vi "DownloadFile.vi"(8 "error in":errorcluster, 11 "Downloader in":refnum<class "Downloader.lvclass">) -> (0 "error out":errorcluster, 3 "Downloader out":refnum<class "Downloader.lvclass">)   [LabVIEW 2014, in "Downloader.lvclass"]
uses:
  Downloader.lvclass
  Downloader.lvclass/Downloader.ctl
  MessageBox/MessageBox.lvclass
  Websocket/Websocket.lvlib
  Download/RasPiDownloader.lvlib
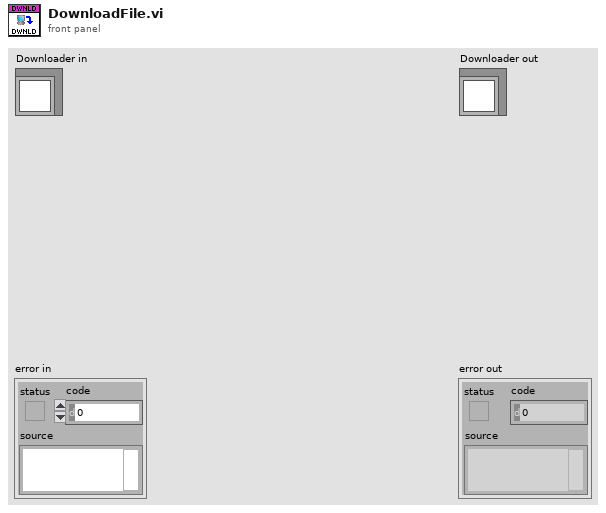
[diagram p1: front panel]
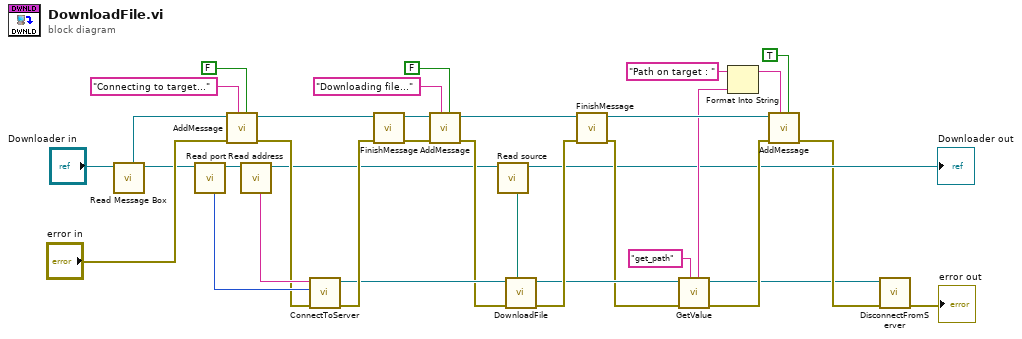
[diagram p0: block diagram]
diagram:
  n1 = call "Read Message Box.vi"("Downloader in"="Downloader in") -> ("Downloader out"=w28:refnum<class "Downloader.lvclass">, "Message Box"=w34:refnum<class "MessageBox.lvclass">)  [unwired: 7 in]
  n2 = call "Read port.vi"("Downloader in"=w28) -> ("Downloader out"=w26:refnum<class "Downloader.lvclass">, "port"=w30:u16)  [unwired: 7 in]
  n3 = call "AddMessage.vi"("add newline"=FALSE, "message"="Connecting to target...", "error in"="error in", "MessageBox in"=w34) -> ("error out"=w27:errorcluster, "MessageBox out"=w25:refnum<class "MessageBox.lvclass">)  [unwired: 4 in]
  n4 = call "Read address.vi"("Downloader in"=w26) -> ("Downloader out"=w16:refnum<class "Downloader.lvclass">, "address"=w29:string)  [unwired: 7 in]
  n5 = call "ConnectToServer.vi"("error in"=w27, "port"=w30, "address"=w29) -> ("error out"=w24:errorcluster, "connection ID"=w19:refnum<k5>)  [unwired: 5 in, 2 out]
  n6 = call "FinishMessage.vi"("error in"=w24, "MessageBox in"=w25) -> ("error out"=w22:errorcluster, "MessageBox out"=w21:refnum<class "MessageBox.lvclass">)  [unwired: 6 in]
  n7 = call "AddMessage.vi"("add newline"=FALSE, "message"="Downloading file...", "error in"=w22, "MessageBox in"=w21) -> ("error out"=w18:errorcluster, "MessageBox out"=w15:refnum<class "MessageBox.lvclass">)  [unwired: 4 in]
  n8 = call "Read source.vi"("Downloader in"=w16) -> ("Downloader out"=→"Downloader out":refnum<class "Downloader.lvclass">, "source"=w17:path)  [unwired: 7 in]
  n9 = call "DownloadFile.vi"("Path"=w17, "error in"=w18, "WebSocket connection"=w19) -> ("error out"=w14:errorcluster, "WebSocket connection out"=w13:refnum<k5>)  [unwired: 5 in]
  n10 = call "FinishMessage.vi"("error in"=w14, "MessageBox in"=w15) -> ("error out"=w11:errorcluster, "MessageBox out"=w9:refnum<class "MessageBox.lvclass">)  [unwired: 6 in]
  n11 = call "GetValue.vi"("cmd"="get_path", "error in"=w11, "connection ID"=w13) -> ("error out"=w10:errorcluster, "connection ID out"=w1:refnum<k5>, "value"=w8:string)  [unwired: 4 in]
  n12 = Format Into String(initial string="Path on target : ", w8) -> (resulting string=w7:string)  [unwired: 2 in, 1 out]
  n13 = call "AddMessage.vi"("add newline"=TRUE, "message"=w7, "error in"=w10, "MessageBox in"=w9) -> ("error out"=w2:errorcluster)  [unwired: 4 in, 1 out]
  n14 = call "DisconnectFromServer.vi"("error in"=w2, "connection ID"=w1) -> ("error out"=→"error out":errorcluster)  [unwired: 7 in]
